vi "[Your Turn Solution] Event-Driven State Machine - Handle Error Locally.vi"() -> ()   [LabVIEW 2020]
uses:
  support/States.ctl
  support/State Machine Data.ctl
  <vilib>/DAQmx/read.llb/DAQmx Read (Analog 2D DBL NChan NSamp).vi
  <vilib>/DAQmx/write.llb/DAQmx Write (Analog DBL 1Chan 1Samp).vi
  <vilib>/DAQmx/create/channels.llb/DAQmx Create Channel (AI-Voltage-Basic).vi
  <vilib>/DAQmx/configure/timing.llb/DAQmx Timing (Sample Clock).vi
  <vilib>/DAQmx/miscellaneous.llb/DAQmx Fill In Error Info.vi
  <vilib>/Utility/file.llb/Write Delimited Spreadsheet (DBL).vi
  <vilib>/DAQmx/create/channels.llb/DAQmx Create Channel (AO-Voltage-Basic).vi
panel:
  in  "AO Voltage Channel":tag="PCI-6221/ao1"
  in  "Generate Stimulus":bool
  out "Threshold exceeded?":bool
  in  "Acquire":bool
  in  "Samples per channel":i32=100
  in  "Sample Rate (Hz)":dbl=1000.0
  in  "AI Voltage Channel":tag="PCI-6221/ai0, PCI-6221/ai2:3"
  in  "Threshold (rms)":dbl=1.0
  in  "Clear":bool
  in  "Exit":bool
  out "Graph":dbl[][](graph)
  # "Analysis"
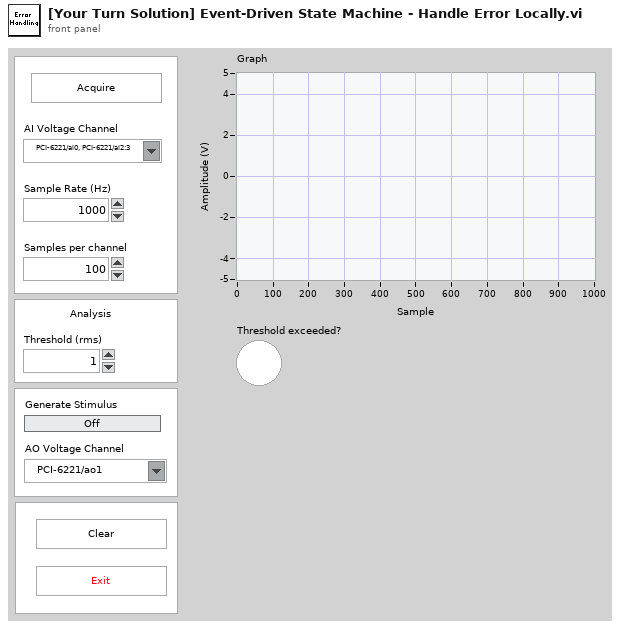
[diagram p1: front panel]
types:
  T1 = typedef "State Machine Data.ctl" = cluster{"Acquisition Data":dbl[][], "Stimulus Value":bool}
  T2 = typedef "States.ctl" = enum16{"Initialize", "Wait for Event", "Acquire", "Analyze", "Log", "Clear", "Update Graph", "Update Stumulus", "Exit"}
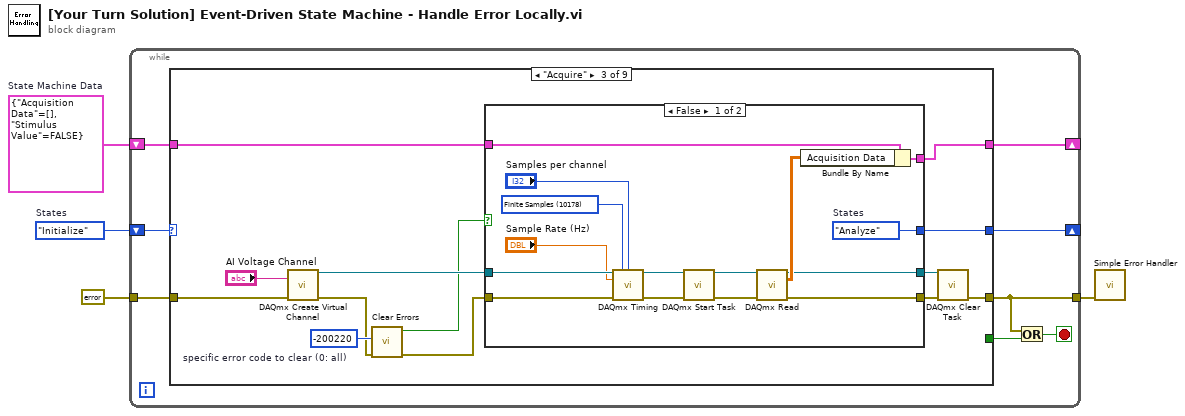
[diagram p0: block diagram]
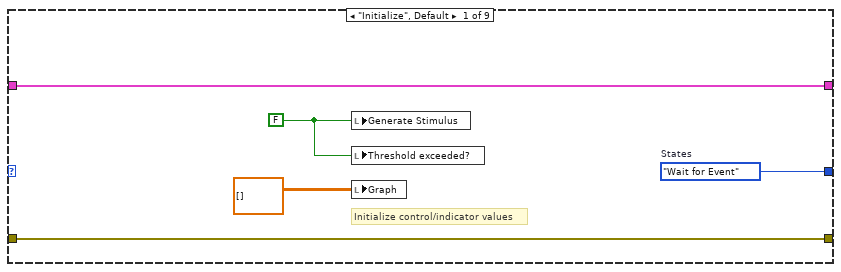
[diagram p2: hidden frame]
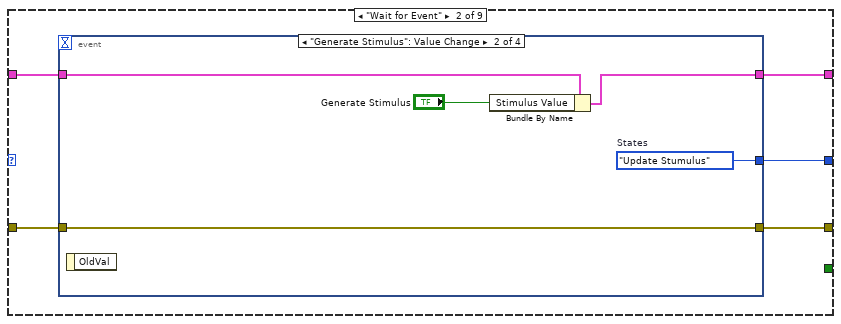
[diagram p3: hidden frame]
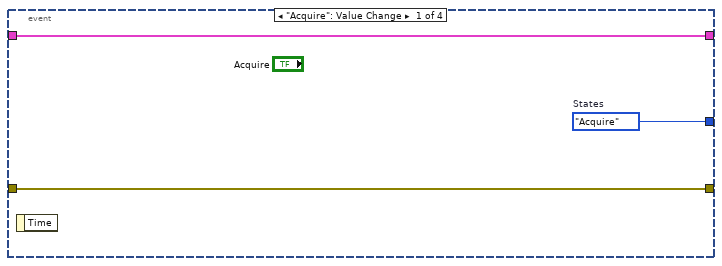
[diagram p4: hidden frame]
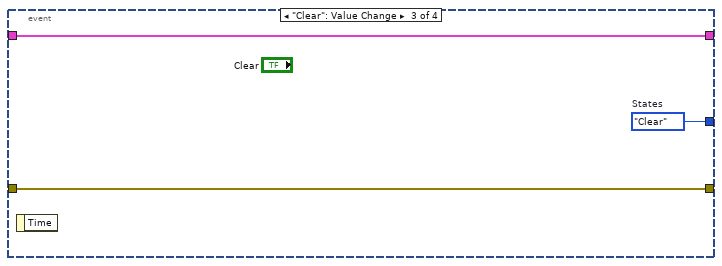
[diagram p5: hidden frame]
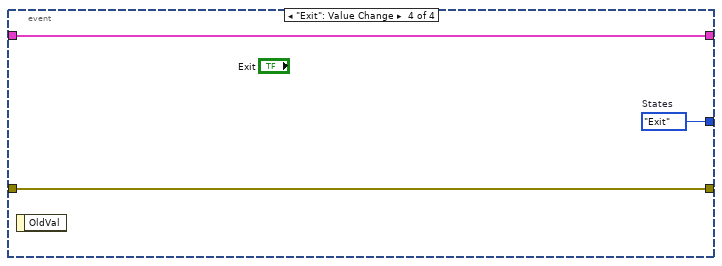
[diagram p6: hidden frame]
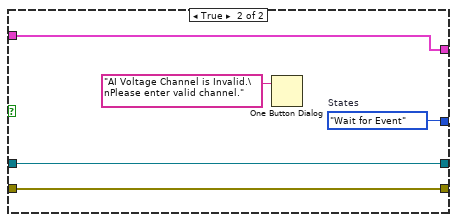
[diagram p7: hidden frame]
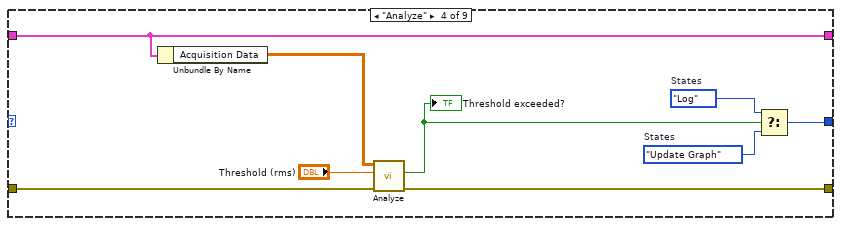
[diagram p8: hidden frame]
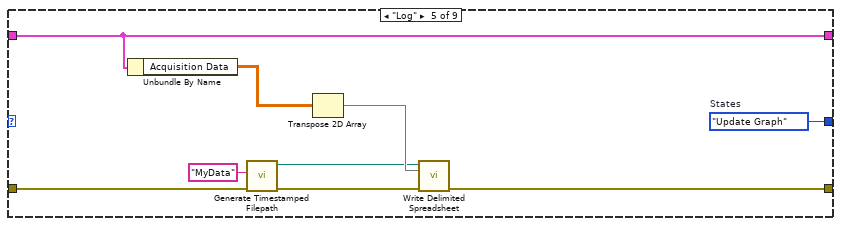
[diagram p9: hidden frame]
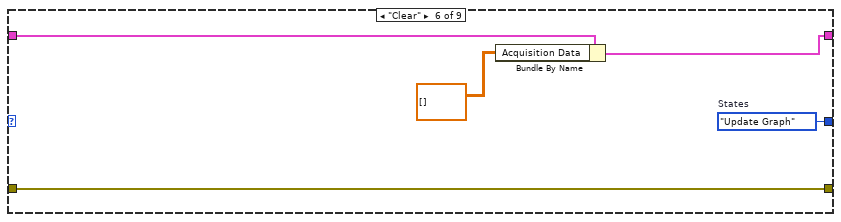
[diagram p10: hidden frame]
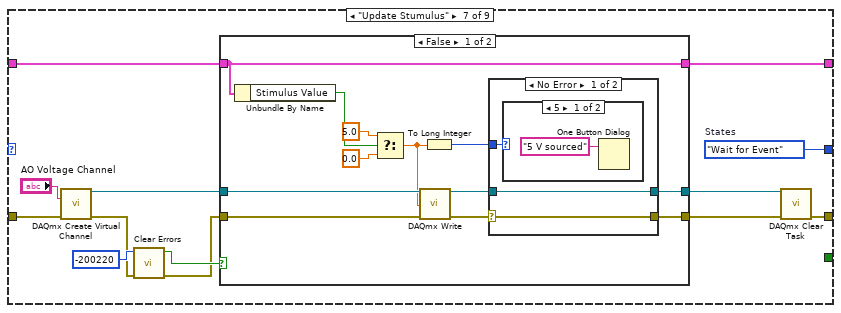
[diagram p11: hidden frame]
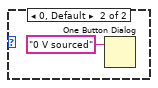
[diagram p12: hidden frame]
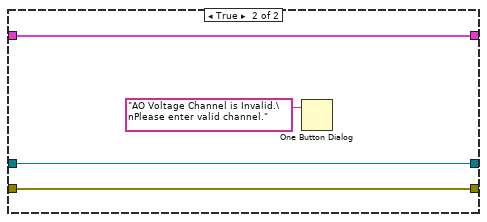
[diagram p14: hidden frame]
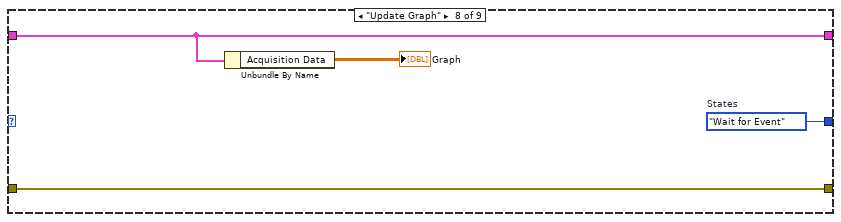
[diagram p15: hidden frame]
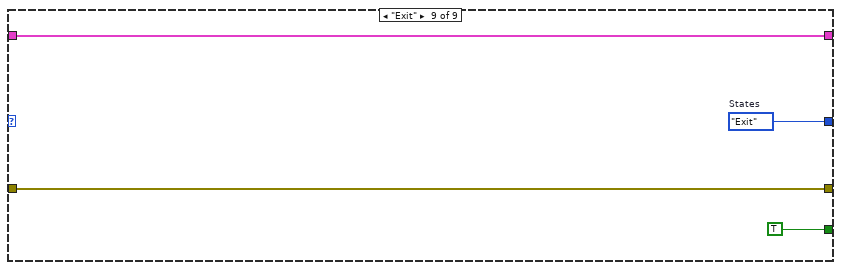
[diagram p16: hidden frame]
diagram:
  w4 = T1 {"Acquisition Data"=[], "Stimulus Value"=FALSE}  # State Machine Data
  w3 = States."Initialize"  # States
  n1 = while {
    tunnel: errorcluster {"status"=FALSE, "code"=0, "source"=""} ("error constant") -> [w11]
    tunnel: [w7] -> w1
    shift-right: [w9] -> _
    shift-left: w4 -> [w10]
    shift-right: [w8] -> _
    shift-left: w3 -> [w12]
    stop <- w6 stop-if-true
    n2 = case shown="\"Acquire\"" w12 {
      tunnel: w11 -> [w17 w20 w49 w77 w86 w92 w102 w131 w135]
      tunnel: [w17 w19 w47 w76 w80 w92 w96 w131 w135] -> w7
      tunnel: [w16 w21 w45 w78 w87 w90 w98 w132 w136] -> w9
      tunnel: w10 -> [w16 w22 w46 w78 w87 w91 w105 w132 w136]
      tunnel: [w15 w18 w41 w72 w79 w88 w94 w130 w133] -> w8
      tunnel: [_ _ _ _ _ _ _ _ TRUE] -> w5
      frame "Initialize", Default {
        w14 = FALSE
        w15 = States."Wait for Event"  # States
        # "Initialize control/indicator values"
        n3 = local write "Generate Stimulus"(w14) -> ()
        n4 = local write "Threshold exceeded?"(w14) -> ()
        n5 = local write "Graph"(dbl[][] []) -> ()
      }
      frame "Wait for Event" {
        n6 = event shown="[1] \"Generate Stimulus\": Value Change" {
          selector: _ -> [_ _ _ _]
          dyn-events: _ -> [_ _ _ _]
          timeout: _ -> [_ _ _ _]
          tunnel: w22 -> [w25 w30 w33 w35]
          tunnel: [w25 w29 w33 w35] -> w21
          tunnel: w20 -> [w24 w26 w32 w36]
          tunnel: [w24 w26 w32 w36] -> w19
          tunnel: [w23 w27 w31 w34] -> w18
          event "Acquire": Value Change {
            w23 = States."Acquire"  # States
            n7 = event-data() -> ()  [unwired: 1 in, 1 out]
          }
          event "Generate Stimulus": Value Change {
            w27 = States."Update Stumulus"  # States
            n8 = event-data() -> ()  [unwired: 1 in, 1 out]
            n9 = Bundle By Name(cluster=w30, "Stimulus Value"="Generate Stimulus") -> (w29:T1)
          }
          event "Clear": Value Change {
            w31 = States."Clear"  # States
            n10 = event-data() -> ()  [unwired: 1 in, 1 out]
          }
          event "Exit": Value Change {
            w34 = States."Exit"  # States
            n11 = event-data() -> ()  [unwired: 1 in, 1 out]
          }
        }
      }
      frame "Acquire" {
        w40 = -200220  # specific error code to clear (0: all)
        n12 = call-poly <vilib>:"DAQmx Create Virtual Channel.vi"("physical channels"="AI Voltage Channel", "error in"=w49) -> ("task out"=w43:refnum<k21>, "error out"=w39:errorcluster)  [unwired: 12 in]
        n13 = call <vilib>:"Clear Errors.vi"("error in (no error)"=w39, "specific error code to clear (0: all)"=w40) -> ("error out"=w38:errorcluster, "specific error cleared?"=w37:bool)  [unwired: 4 in]
        n14 = case shown="False" w37 {
          tunnel: w38 -> [w64 w67]
          tunnel: [w61 w67] -> w48
          tunnel: w46 -> [w60 w69]
          tunnel: [w59 w69] -> w45
          tunnel: w43 -> [w55 w68]
          tunnel: [w52 w68] -> w42
          tunnel: [w50 w66] -> w41
          frame False {
            w50 = States."Analyze"  # States
            w58 = 10178 items=["Finite Samples"=10178, "Continuous Samples"=10123, "Hardware Timed Single Point"=12522] ("sample mode")
            n15 = call-poly <vilib>:"DAQmx Timing.vi"("task/channels in"=w55, "sample mode"=w58, "samples per channel"="Samples per channel", "rate"="Sample Rate (Hz)", "error in"=w64) -> ("task out"=w54:refnum<k21>, "error out"=w63:errorcluster)  [unwired: 9 in]
            n16 = call <vilib>:"DAQmx Start Task.vi"("task/channels in"=w54, "error in"=w63) -> ("task out"=w53:refnum<k21>, "error out"=w62:errorcluster)  [unwired: 12 in]
            n17 = call-poly <vilib>:"DAQmx Read.vi"("task/channels in"=w53, "error in"=w62) -> ("task out"=w52:refnum<k21>, "data"=w56:dbl[][], "error out"=w61:errorcluster)  [unwired: 11 in]
            n18 = Bundle By Name(cluster=w60, "Acquisition Data"=w56) -> (w59:T1)
          }
          frame True {
            w66 = States."Wait for Event"  # States
            n19 = One Button Dialog(message="AI Voltage Channel is Invalid.\nPlease enter valid channel.") -> ()  [unwired: 1 in, 1 out]
          }
        }
        n20 = call <vilib>:"DAQmx Clear Task.vi"("task in"=w42, "error in"=w48) -> ("error out"=w47:errorcluster)  [unwired: 13 in]
      }
      frame "Analyze" {
        w73 = States."Update Graph"  # States
        w74 = States."Log"  # States
        n21 = Unbundle By Name(w78) -> ("Acquisition Data"=w75:dbl[][])
        n22 = call "Analyze.vi"("Error In"=w77, "Treshold (rms)"="Threshold (rms)", "N-Channel Data (2D DBL)"=w75) -> ("Error Out"=w76:errorcluster, "Threshold exceeded?"=w70:bool)  [unwired: 5 in, 2 out]
        "Threshold exceeded?" <- w70
        n23 = Select(t=w74, s=w70, f=w73) -> (s? t:f=w72:T2)
      }
      frame "Log" {
        w79 = States."Update Graph"  # States
        n24 = Unbundle By Name(w87) -> ("Acquisition Data"=w84:dbl[][])
        n25 = call "Generate Timestamped Filepath.vi"("Error In"=w86, "appended filename"="MyData") -> ("Error Out"=w81:errorcluster, "timestamped relative filepath"=w82:path)  [unwired: 8 in]
        n26 = Transpose 2D Array(2D array=w84) -> (transposed array=w83:dbl[][])
        n27 = call-poly <vilib>:"Write Delimited Spreadsheet.vi"("file path (dialog if empty)"=w82, "2D data"=w83, "error in (no error)"=w81) -> ("error out"=w80:errorcluster)  [unwired: 11 in, 1 out]
      }
      frame "Clear" {
        w88 = States."Update Graph"  # States
        n28 = Bundle By Name(cluster=w91, "Acquisition Data"=dbl[][] []) -> (w90:T1)
      }
      frame "Update Stumulus" {
        w94 = States."Wait for Event"  # States
        n29 = call-poly <vilib>:"DAQmx Create Virtual Channel.vi"("physical channels"="AO Voltage Channel", "error in"=w102) -> ("task out"=w104:refnum<k21>, "error out"=w100:errorcluster)  [unwired: 12 in]
        n30 = call <vilib>:"Clear Errors.vi"("error in (no error)"=w100, "specific error code to clear (0: all)"=-200220) -> ("error out"=w93:errorcluster, "specific error cleared?"=w99:bool)  [unwired: 4 in]
        n31 = case shown="False" w99 {
          tunnel: w105 -> [w110 w127]
          tunnel: w104 -> [w115 w126]
          tunnel: [w106 w125] -> w97
          tunnel: w93 -> [w111 w125]
          tunnel: [w110 w127] -> w98
          tunnel: [w108 w126] -> w95
          frame False {
            n32 = Unbundle By Name(w110) -> ("Stimulus Value"=w112:bool)
            n33 = Select(t=5.0, s=w112, f=0.0) -> (s? t:f=w114:dbl)
            n34 = call-poly <vilib>:"DAQmx Write.vi"("task/channels in"=w115, "data"=w114, "error in"=w111) -> ("task out"=w109:refnum<k21>, "error out"=w107:errorcluster)  [unwired: 10 in, 1 out]
            n35 = To Long Integer(number=w114) -> (32bit integer=w113:i32)
            n36 = case shown="No Error" w107 {
              selector: w107 -> [w118 w124]
              tunnel: w113 -> [w120 _]
              tunnel: w109 -> [w119 w123]
              tunnel: [w119 w123] -> w108
              tunnel: [w118 w124] -> w106
              frame No Error {
                n37 = case shown="5" w120 {
                  frame 5 {
                    n38 = One Button Dialog(message="5 V sourced") -> ()  [unwired: 1 in, 1 out]
                  }
                  frame 0, Default {
                    n39 = One Button Dialog(message="0 V sourced") -> ()  [unwired: 1 in, 1 out]
                  }
                }
              }
              frame Error {
              }
            }
          }
          frame True {
            n40 = One Button Dialog(message="AO Voltage Channel is Invalid.\nPlease enter valid channel.") -> ()  [unwired: 1 in, 1 out]
          }
        }
        n41 = call <vilib>:"DAQmx Clear Task.vi"("task in"=w95, "error in"=w97) -> ("error out"=w96:errorcluster)  [unwired: 13 in]
      }
      frame "Update Graph" {
        w130 = States."Wait for Event"  # States
        n42 = Unbundle By Name(w132) -> ("Acquisition Data"=→"Graph":dbl[][])
      }
      frame "Exit" {
        w133 = States."Exit"  # States
      }
    }
    n43 = Or(x=w7, y=w5) -> (x .or. y?=w6:bool)
  }
  n44 = call <vilib>:"Simple Error Handler.vi"("error in (no error)"=w1) -> ()  [unwired: 4 in, 5 out]
